vi "Calculate speed using distance.vi"(0 "Distance":dbl, 5 "Min dist for movement":dbl=100.0, 7 "Distance for max speed":dbl=500.0, 9 "Min absolute speed":dbl, 11 "error in":errorcluster, 12 "Trans spd multiplier":dbl=1.0) -> (4 "Trans spd percentage (0 to 1)":dbl, 14 "Trans spd out":dbl, 15 "error out":errorcluster)   [LabVIEW 2016]
panel:
  # "Linear scaling system for determining speed\nAlternatives: Using a log function or other non-linear scaling method"
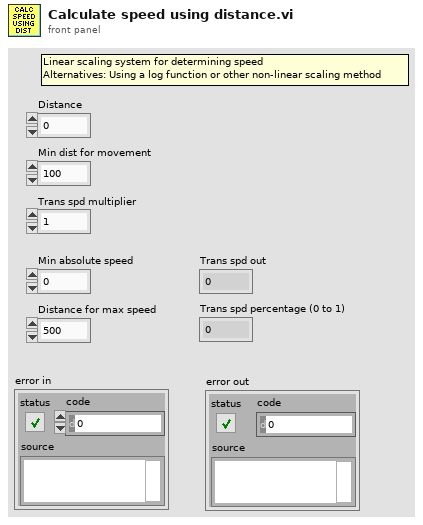
[diagram p1: front panel]
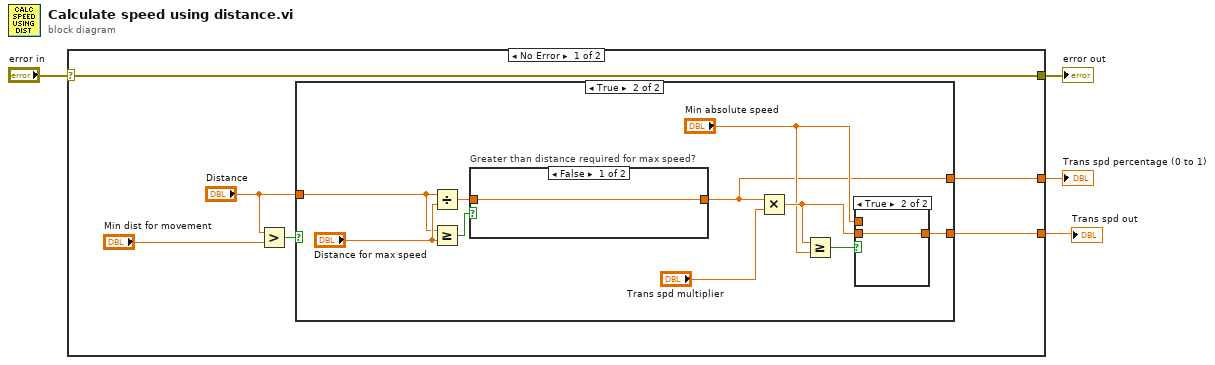
[diagram p0: block diagram]
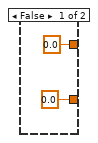
[diagram p2: hidden frame]
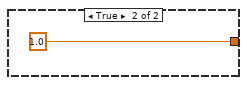
[diagram p4: hidden frame]
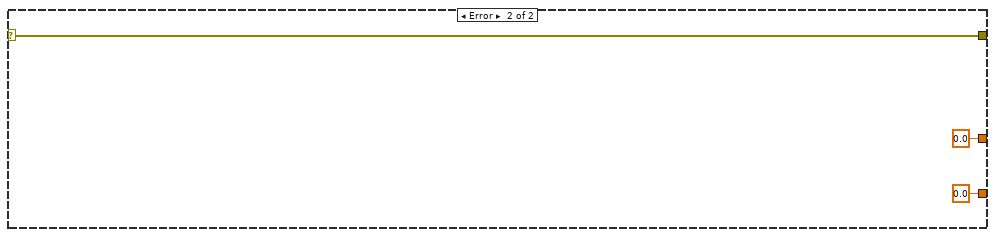
[diagram p5: hidden frame]
diagram:
  n1 = case shown="No Error" "error in" {
    selector: "error in" -> [w7 w29]
    tunnel: [w7 w29] -> w3
    tunnel: [w6 0.0 ("Min absolute speed")] -> w2
    tunnel: [w5 0.0 ("speed out")] -> w1
    frame No Error {
      n2 = Greater?(x="Distance", y="Min dist for movement") -> (0:w8:bool)
      n3 = case shown="True" w8 {
        tunnel: "Distance" -> [_ w15]
        tunnel: [0.0 ("Min absolute speed") w14] -> w6
        tunnel: [0.0 ("speed out") w13] -> w5
        frame False {
        }
        frame True {
          n4 = Divide(x=w15, y="Distance for max speed") -> (x/y=w20:dbl)
          n5 = Greater Or Equal?(x=w15, y="Distance for max speed") -> (x >= y?=w21:bool)
          n6 = case "Greater than distance required for max speed?" shown="False" w21 {
            tunnel: [w25 1.0 ("speed out")] -> w13
            tunnel: w20 -> [w25 _]
            frame False {
            }
            frame True {
            }
          }
          n7 = Multiply(x=w13, y="Trans spd multiplier") -> (x*y=w17:dbl)
          n8 = Greater Or Equal?(x=w17, y="Min absolute speed") -> (x >= y?=w19:bool)
          n9 = case shown="True" w19 {
            tunnel: w17 -> [_ w24]
            tunnel: [w23 w24] -> w14
            tunnel: "Min absolute speed" -> [w23 _]
            frame False {
            }
            frame True {
            }
          }
        }
      }
    }
    frame Error {
    }
  }
  "error out" <- w3
  "Trans spd out" <- w2
  "Trans spd percentage (0 to 1)" <- w1
